vi "Channel ID to Mode ID.vi"(9 "TIRF Mode N":T1, 10 "Widefield mode?":bool, 11 "Channel ID":i8) -> (3 "Mode ID":i8)   [LabVIEW 2018]
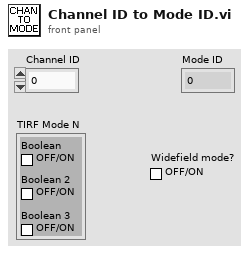
[diagram p1: front panel]
types:
  T1 = cluster{"Boolean":bool, "Boolean 2":bool, "Boolean 3":bool}
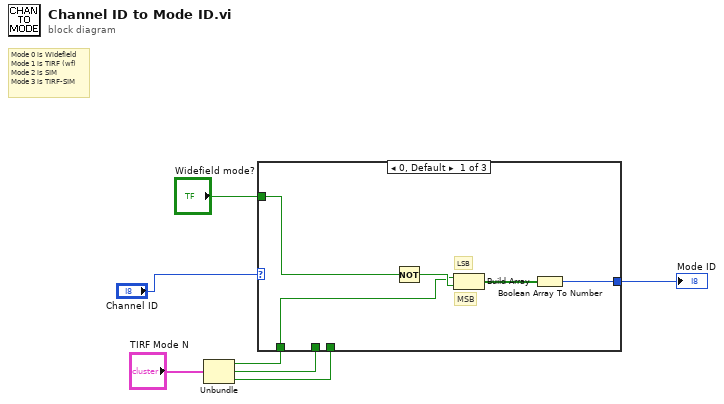
[diagram p0: block diagram]
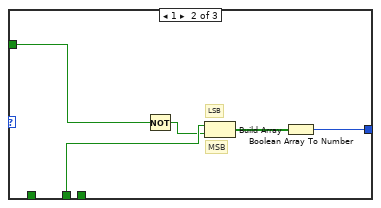
[diagram p2: hidden frame]
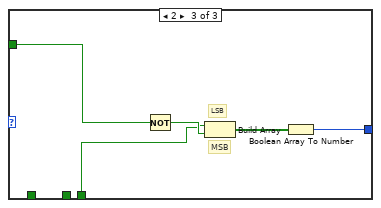
[diagram p3: hidden frame]
diagram:
  # "Mode 0 is Widefield\nMode 1 is TIRF (wf)\nMode 2 is SIM\nMode 3 is TIRF-SIM"
  n1 = Unbundle("TIRF Mode N") -> ("Boolean"=w5:bool, "Boolean 2"=w4:bool, "Boolean 3"=w3:bool)
  n2 = case shown="0, Default" "Channel ID" {
    tunnel: w5 -> [w8 _ _]
    tunnel: w4 -> [_ w14 _]
    tunnel: w3 -> [_ _ w18]
    tunnel: "Widefield mode?" -> [w11 w16 w21]
    tunnel: [w10 w15 w20] -> w1
    frame 0, Default {
      # "MSB"
      # "LSB"
      n3 = Not(x=w11) -> (.not. x?=w9:bool)
      n4 = Build Array(w8, w9) -> (w12:bool[])
      n5 = Boolean Array To Number(Boolean array=w12) -> (number=w10:u32)
    }
    frame 1 {
      # "MSB"
      # "LSB"
      n6 = Not(x=w16) -> (.not. x?=w13:bool)
      n7 = Build Array(w14, w13) -> (w17:bool[])
      n8 = Boolean Array To Number(Boolean array=w17) -> (number=w15:u32)
    }
    frame 2 {
      # "MSB"
      # "LSB"
      n9 = Not(x=w21) -> (.not. x?=w19:bool)
      n10 = Build Array(w18, w19) -> (w22:bool[])
      n11 = Boolean Array To Number(Boolean array=w22) -> (number=w20:u32)
    }
  }
  "Mode ID" <- w1
